vi "JayDrive.vi"(5 "StraightDrive":bool, 7 "SpeedControl":bool, 8 "error in (no error)":errorcluster, 9 "Right Axis":dbl, 10 "Left Axis":dbl, 11 "RobotDriveDevRef":T1={"DevStatus"={"status"=FALSE, "code"=0, "source"=""}, "Motors[]"=[], "Square Inputs"=FALSE, "Max Output"=1.0, "Isochronous"=FALSE}) -> (0 "error out":errorcluster, 3 "RobotDriveDevRef":T1={"DevStatus"={"status"=FALSE, "code"=0, "source"=""}, "Motors[]"=[], "Square Inputs"=FALSE, "Max Output"=1.0, "Isochronous"=FALSE})   [LabVIEW 2011]
uses:
  <vilib>/Rock Robotics/WPI/RobotDrive/WPI_RobotDriveDevRef.ctl
  <vilib>/Rock Robotics/WPI/MotorControl/WPI_MotorControlDeviceRef.ctl
  <vilib>/Rock Robotics/SystemInterfaces/Typedef/FPGA_TypedefDigitalModule.ctl
  <vilib>/Rock Robotics/SystemInterfaces/DIO/FPGA_DIOPWMChannel.ctl
  <vilib>/Rock Robotics/WPI/PWM/WPI_PWMDeadband.ctl
  <vilib>/Rock Robotics/WPI/CAN/Jaguar/SubVIs/WPI_CANJaguar_ControlMode.ctl
  <vilib>/Rock Robotics/WPI/PWM/WPI_PWMTransform_ConPane.ctl
  Robot Global Data.vi
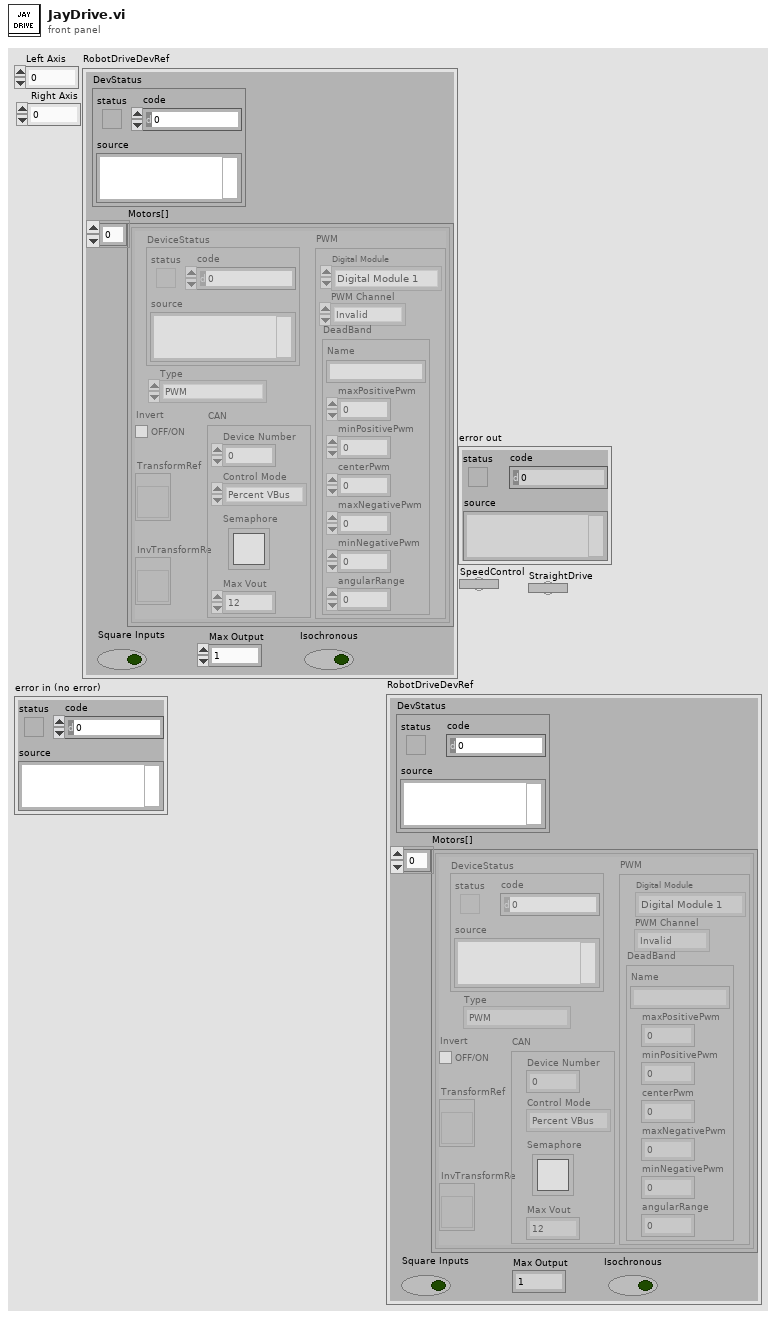
[diagram p1: front panel]
types:
  T1 = typedef "WPI_RobotDriveDevRef.ctl" = cluster{"DevStatus":errorcluster, "Motors[]":T2[], "Square Inputs":bool, "Max Output":dbl, "Isochronous":bool}
  T2 = typedef "WPI_MotorControlDeviceRef.ctl" = cluster{"DeviceStatus":errorcluster, "Type":enum16{"PWM", "CAN"}, "PWM":cluster{"Digital Module":T3, "PWM Channel":T4, "DeadBand":T5}, "CAN":cluster{"Device Number":u8, "Control Mode":T6, "Semaphore":T7, "Max Vout":dbl}, "Invert":bool, "TransformRef":T8, "InvTransformRef":T8}
  T3 = typedef "FPGA_TypedefDigitalModule.ctl" = enum16{"Digital Module 1", "Digital Module 2"}
  T4 = typedef "FPGA_DIOPWMChannel.ctl" = enum8{"PWM 1", "PWM 2", "PWM 3", "PWM 4", "PWM 5", "PWM 6", "PWM 7", "PWM 8", "PWM 9", "PWM 10", "Invalid"}
  T5 = typedef "WPI_PWMDeadband.ctl" = cluster{"Name":string, "maxPositivePwm":i32, "minPositivePwm":i32, "centerPwm":i32, "maxNegativePwm":i32, "minNegativePwm":i32, "angularRange":u16}
  T6 = typedef "WPI_CANJaguar_ControlMode.ctl" = enum8{"Percent VBus", "Current", "Speed", "Position", "Voltage"}
  T7 = typedef "Semaphore RefNum" = refnum<k1>
  T8 = typedef "WPI_PWMTransform_ConPane.ctl" = refnum<vi>
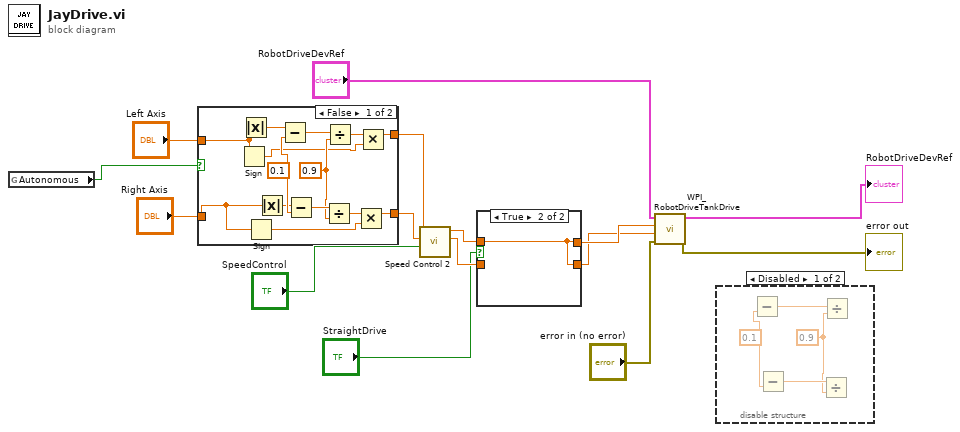
[diagram p0: block diagram]
diagram:
  n1 = global read "Robot Global Data.vi" "Autonomous"() -> (w3:bool)
  n2 = case shown="False" w3 {
    tunnel: "Left Axis" -> [w17 w31]
    tunnel: "Right Axis" -> [w21 w30]
    tunnel: [w20 w30] -> w2
    tunnel: [w18 w31] -> w1
    frame False {
      w26 = 0.9 ("y")
      w29 = 0.1 ("y")
      n3 = Sign(1:w17) -> (0:w16:dbl)
      n4 = Absolute Value(x=w17) -> (abs(x)=w23:dbl)
      n5 = Sign(1:w21) -> (0:w19:dbl)
      n6 = Absolute Value(x=w21) -> (abs(x)=w22:dbl)
      n7 = Subtract(x=w23, y=w29) -> (x-y=w28:dbl)
      n8 = Subtract(x=w22, y=w29) -> (x-y=w27:dbl)
      n9 = Divide(x=w27, y=w26) -> (x/y=w25:dbl)
      n10 = Divide(x=w28, y=w26) -> (x/y=w24:dbl)
      n11 = Multiply(x=w25, y=w19) -> (x*y=w20:dbl)
      n12 = Multiply(x=w24, y=w16) -> (x*y=w18:dbl)
    }
    frame True {
    }
  }
  n13 = call "Speed Control 2.vi"("Boolean"="SpeedControl", "Right Axis"=w2, "Left Axis"=w1) -> ("Right motor"=w9:dbl, "Left Motor"=w10:dbl)  [unwired: 7 in]
  n14 = case shown="True" "StraightDrive" {
    tunnel: [w33 w34] -> w8
    tunnel: w10 -> [w33 w34]
    tunnel: [w32 w34] -> w7
    tunnel: w9 -> [w32 _]
    frame False {
    }
    frame True {
    }
  }
  n15 = call <vilib>:"WPI_RobotDriveTankDrive.vi"("error in (no error)"="error in (no error)", "Right axis value"=w7, "Left axis value"=w8, "RobotDriveDevRef"="RobotDriveDevRef") -> ("error out"=→"error out":errorcluster, "RobotDriveDevRef"=→"RobotDriveDevRef":T1)  [unwired: 6 in]
  n16 = disable-structure shown="Disabled" {
    frame Disabled {
      w35 = 0.9 ("y")
      w38 = 0.1 ("y")
      n17 = Subtract(y=w38) -> (x-y=w37:dbl)  [unwired: 1 in]
      n18 = Subtract(y=w38) -> (x-y=w36:dbl)  [unwired: 1 in]
      n19 = Divide(x=w36, y=w35) -> ()  [unwired: 1 out]
      n20 = Divide(x=w37, y=w35) -> ()  [unwired: 1 out]
    }
    frame Enabled {
    }
  }
